vi "2xMonitor.vi"   [LabVIEW 2016]
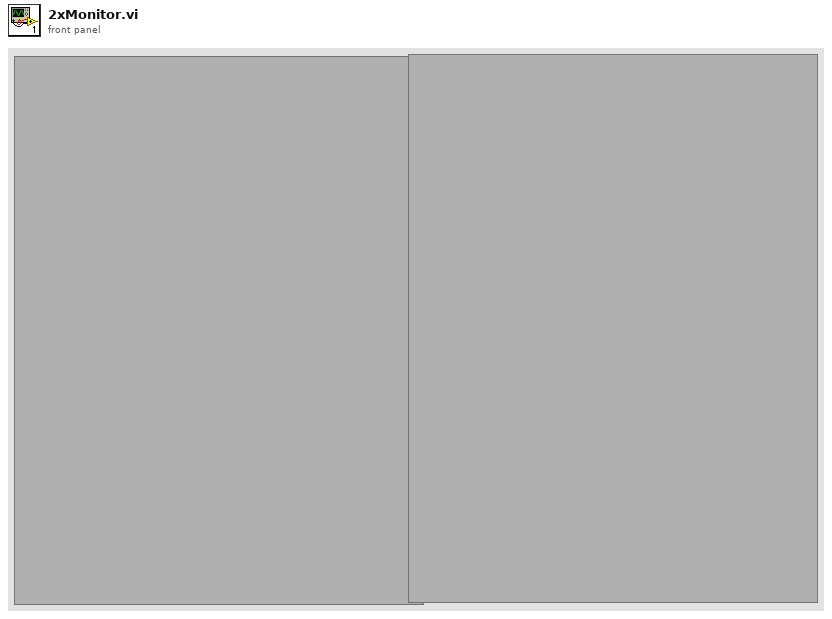
[diagram p1: front panel]
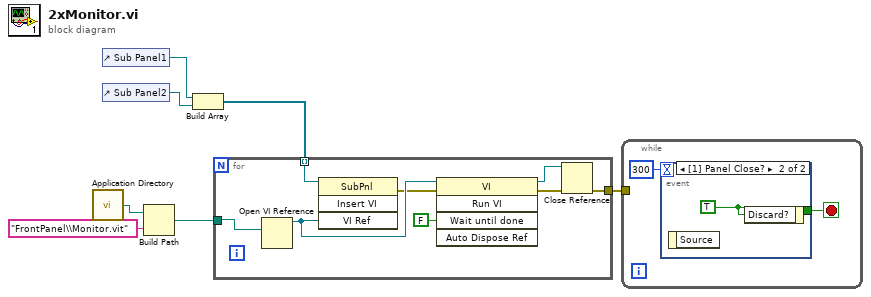
[diagram p0: block diagram]
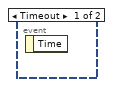
[diagram p2: hidden frame]
diagram:
  n1 = call <vilib>:"Application Directory.vi"() -> ("Application Directory"=w5:path)
  n2 = control-ref of="Sub Panel1"() -> (w7:refnum<vi>)
  n3 = control-ref of="Sub Panel2"() -> (w6:refnum<vi>)
  n4 = Build Path(base path=w5, name or relative path="FrontPanel\\Monitor.vit") -> (appended path=w4:path)
  n5 = Build Array(w7, w6) -> (w1:refnum<vi>[])
  n6 = for {
    tunnel: w4 -> [w11]
    tunnel: w1 -> [w15] mode=indexing
    tunnel: [w8] -> w2
    n7 = Open VI Reference(vi path=w11) -> (vi reference=w14:refnum<vi>)  [unwired: 5 in, 1 out]
    n8 = invoke on="Invoke Node" class="SubPnl" method="Insert VI"(reference=w15, "VI Ref"=w14) -> (error out=w13:errorcluster)  [unwired: 2 in, 3 out]
    n9 = invoke class="VI" method="Run VI"(reference=w14, error in=w13, "Wait until done"=FALSE ("Wait Until Done")) -> (reference out=w10:refnum<vi>, error out=w9:errorcluster)  [unwired: 2 in, 3 out]
    n10 = Close Reference(reference=w10, error in (no error)=w9) -> (error out=w8:errorcluster)
  }
  n11 = while {
    tunnel: w2 -> [_]
    stop <- w17 stop-if-true
    n12 = event shown="[1] Panel Close?" {
      selector: _ -> [_ _]
      dyn-events: _ -> [_ _]
      timeout: 300 -> [_ _]
      tunnel: [_ w18] -> w17
      event Timeout {
        n13 = event-data() -> ()  [unwired: 1 in, 1 out]
      }
      event Panel Close? {
        w18 = TRUE ("stop")
        n14 = event-data() -> ()  [unwired: 1 in, 1 out]
        n15 = event-data("Discard?"=w18) -> ()  [unwired: 1 in, 1 out]
      }
    }
  }
